vi "InstallFPP.vi"() -> ()   [LabVIEW 2014, in "Installer.lvlib"]
uses:
  Installer.lvlib
  ProgressMessage.ctl
panel:
  out "Progress":i8(slide) scale=0.0..100.0
  out "error out":errorcluster
  in  "error in (no error)":errorcluster
  out "Status":string
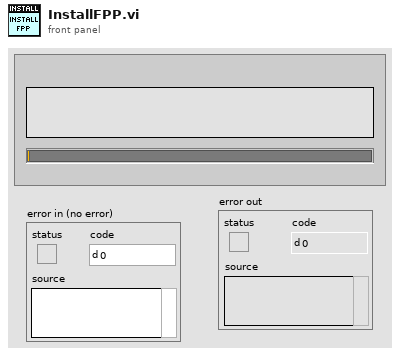
[diagram p1: front panel]
types:
  T1 = typedef "Installer.lvlib/ProgressMessage.ctl" = cluster{"Task":string, "Progress":i8}
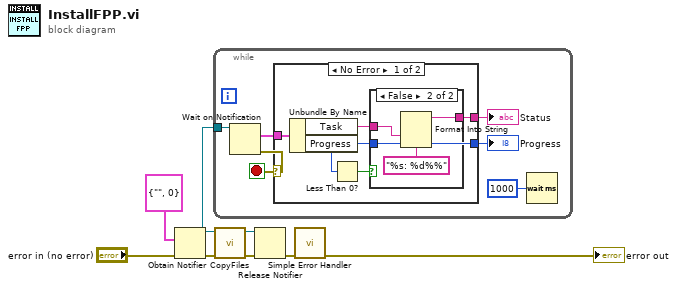
[diagram p0: block diagram]
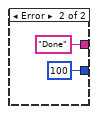
[diagram p3: hidden frame]
diagram:
  n1 = Obtain Notifier(notification data type=T1 {"Task"="", "Progress"=0}, error in (no error)="error in (no error)") -> (notifier out=w7:refnum<notifier>, error out=w6:errorcluster)  [unwired: 2 in, 1 out]
  n2 = while {
    tunnel: w7 -> [w14]
    stop <- w10 stop-if-true
    n3 = Wait on Notification(notifier=w14) -> (notification=w13:T1, error out=w10:errorcluster)  [unwired: 3 in, 2 out]
    n4 = case shown="No Error" w10 {
      tunnel: w13 -> [w19 _]
      tunnel: [w16 "Done" ("Task")] -> w12
      tunnel: [w15 i8 100 ("Progress")] -> w11
      frame No Error {
        n5 = Unbundle By Name(w19) -> ("Task"=w18:string, "Progress"=w15:i8)
        n6 = Less Than 0?(x=w15) -> (x < 0?=w17:bool)
        n7 = case shown="False" w17 {
          tunnel: w18 -> [w20 w24]
          tunnel: w15 -> [_ w22]
          tunnel: [w20 w21] -> w16
          frame True {
          }
          frame False {
            n8 = Format Into String(format string="%s: %d%%", w24, w22) -> (resulting string=w21:string)  [unwired: 2 in, 1 out]
          }
        }
      }
      frame Error {
      }
    }
    "Status" <- w12
    "Progress" <- w11
    n9 = Wait (ms)(milliseconds to wait=u32 1000) -> ()  [unwired: 1 out]
  }
  n10 = call "CopyFiles.vi"("error in (no error)"=w6, "Progress notifier"=w7) -> ("error out"=w2:errorcluster, "Progress notifier dup"=w1:refnum<notifier>)  [unwired: 8 in]
  n11 = Release Notifier(notifier=w1, error in (no error)=w2) -> (error out=w4:errorcluster)  [unwired: 1 in, 2 out]
  n12 = call <vilib>:"Simple Error Handler.vi"("error in (no error)"=w4) -> ("error out"=→"error out":errorcluster)  [unwired: 4 in, 4 out]
